vi "svfa_Check Data Valid [FFT] (N Ch).vi"(0 "scaled signals":waveform(dbl)[](array[waveform]), 2 "restart averaging (F)":bool, 7 "window":T2=1 items=["None"=0, "Hanning"=1, "Hamming"=2, "Blackman-Harris"=3, "Exact Blackman"=4, "Blackman"=5, "Flat Top"=6, "4 Term B-Harris "=7, "7 Term B-Harris"=8, "Low Sidelobe"=9, "Force"=64, "Exponential"=65, "Blackman Nuttall"=11, "Triangle"=30, "Bartlett-Hanning"=31, "Bohman"=32, "Parzen"=33, "Welch"=34, "Kaiser"=60, "Dolph-Chebyshev"=61, "Gaussian"=62], 9 "averaging parameters":T1={"averaging mode"=enum."No averaging", "weighting mode"=enum."Linear", "number of averages"=10, "linear mode"=enum."Auto restart"}, 11 "error in (no error)":errorcluster) -> (3 "restart averaging":bool, 4 "dup scaled signals":waveform(dbl)[](array[waveform]), 8 "dup window":T2=1 items=["None"=0, "Hanning"=1, "Hamming"=2, "Blackman-Harris"=3, "Exact Blackman"=4, "Blackman"=5, "Flat Top"=6, "4 Term B-Harris "=7, "7 Term B-Harris"=8, "Low Sidelobe"=9, "Force"=64, "Exponential"=65, "Blackman Nuttall"=11, "Triangle"=30, "Bartlett-Hanning"=31, "Bohman"=32, "Parzen"=33, "Welch"=34, "Kaiser"=60, "Dolph-Chebyshev"=61, "Gaussian"=62], 10 "dup averaging parameters":T1, 15 "error out":errorcluster)   [LabVIEW 2017]
doc: "returns errors on invalid parameters \nchecks for property changes (such as dt) and configuration changes (such as window), returns restart = TRUE on change"
uses:
  <vilib>/addons/_NISVFA/_Shared subVIs/Controls/svc_Window.ctl
  <vilib>/addons/_NISVFA/_Shared subVIs/Common/svc_Check for Waveform Parameter Continuity (no state).vi
  <vilib>/addons/_NISVFA/_Shared subVIs/Common/svc_Get SV Channel Info.vi
  <vilib>/addons/_NISVFA/_Shared subVIs/Common/svc_Engineering Units to Unit Label.vi
  <vilib>/addons/_NISVFA/_Shared subVIs/Common/svc_Unit Label to Engineering Units.vi
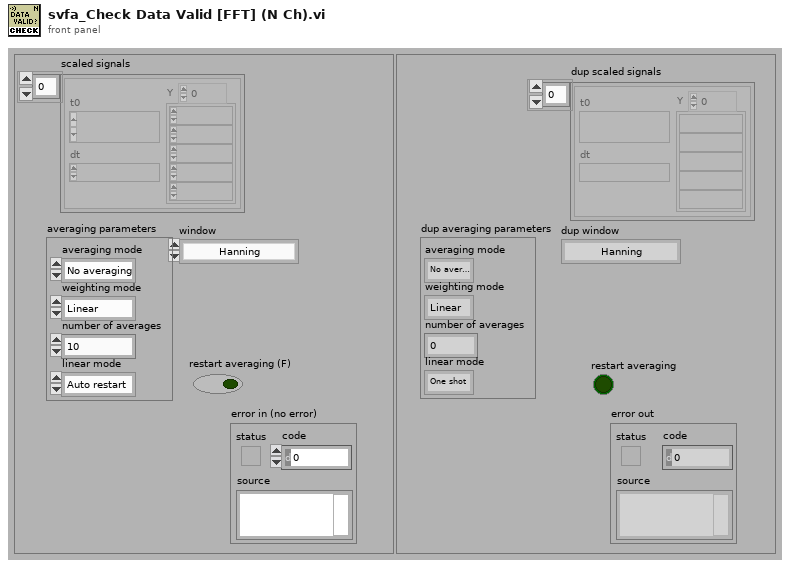
[diagram p1: front panel]
types:
  T1 = cluster{"averaging mode":enum16{"No averaging", "Vector averaging", "RMS averaging", "Peak hold"}, "weighting mode":enum16{"Linear", "Exponential"}, "number of averages":u32, "linear mode":enum16{"One shot", "Auto restart"}}
  T2 = typedef "svc_Window.ctl" = u32
  T3 = cluster{"dt equal":bool, "array length equal":bool, "number channels change":bool}
  T4 = cluster{"dt":bool, "t0 continuity":bool, "array length":bool, "channel info":bool, "name":bool}
  T5 = enum16{"No averaging", "Vector averaging", "RMS averaging", "Peak hold"}
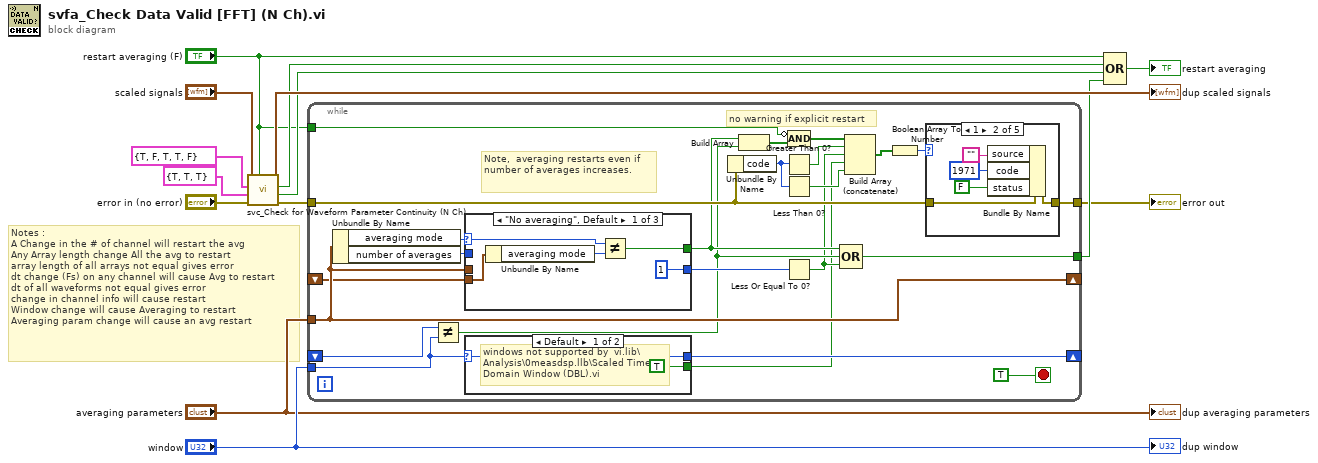
[diagram p0: block diagram]
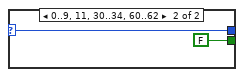
[diagram p2: hidden frame]
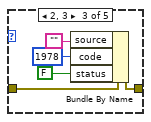
[diagram p4: hidden frame]
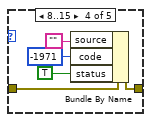
[diagram p5: hidden frame]
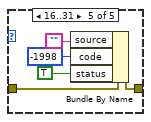
[diagram p6: hidden frame]
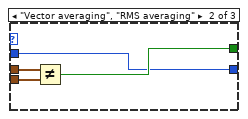
[diagram p7: hidden frame]
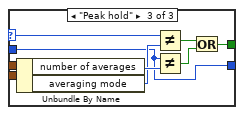
[diagram p8: hidden frame]
diagram:
  # "Notes : \nA Change in the # of channel will restart the avg\nAny Array length change All the avg to restart\narray length of all arrays not equal gives error\ndt change (Fs) on any channel will cause Avg to restart\ndt of all waveforms not equal gives error\nchange in channel info will cause restart\nWindow change will cause Averaging to restart\nAveraging param change will cause an avg restart"
  n1 = call <vilib>:"svc_Check for Waveform Parameter Continuity (N Ch).vi"("restart averaging (F)"="restart averaging (F)", "error in (no error)"="error in (no error)", "checks for multichannel parameters"=T3 {"dt equal"=TRUE, "array length equal"=TRUE, "number channels change"=TRUE}, "checks for channel parameter change"=T4 {"dt"=TRUE, "t0 continuity"=FALSE, "array length"=TRUE, "channel info"=TRUE, "name"=FALSE}, "scaled signal(s)"="scaled signals") -> ("error out"=w6:errorcluster, "multichannel parameter changed"=w9:bool, "waveform parameter changed"=w10:bool, "dup scaled signal(s)"=→"dup scaled signals":waveform(dbl)[])  [unwired: 3 out]
  n2 = while {
    tunnel: w6 -> [w23]
    tunnel: "restart averaging (F)" -> [w27]
    shift-right: [w16] -> _
    shift-left: _ -> [w37]
    tunnel: "window" -> [w17]
    shift-right: [w29] -> _
    shift-left: _ -> [w28]
    tunnel: "averaging parameters" -> [w29]
    tunnel: [w18] -> w4
    tunnel: [w22] -> w3
    stop <- TRUE stop-if-true
    # "Note,  averaging restarts even if number of averages increases."
    # "no warning if explicit restart"
    n3 = Unbundle By Name(w29) -> ("averaging mode"=w36:T5, "number of averages"=w35:u32)
    n4 = Not Equal?(x=w37, y=w17) -> (x != y?=w20:bool)
    n5 = case shown="\"No averaging\", Default" w36 {
      selector: w36 -> [w65 _ w76]
      tunnel: w29 -> [_ w71 _]
      tunnel: w28 -> [w68 w72 w75]
      tunnel: [w67 w70 w77] -> w21
      tunnel: w35 -> [_ w69 w73]
      tunnel: [u32 1 ("number of averages") w69 w73] -> w30
      frame "No averaging", Default {
        n6 = Unbundle By Name(w68) -> ("averaging mode"=w66:T5)
        n7 = Not Equal?(x=w65, y=w66) -> (x != y?=w67:bool)
      }
      frame "Vector averaging", "RMS averaging" {
        n8 = Not Equal?(x=w71, y=w72) -> (x != y?=w70:bool)
      }
      frame "Peak hold" {
        n9 = Unbundle By Name(w75) -> ("number of averages"=w80:u32, "averaging mode"=w74:T5)
        n10 = Not Equal?(x=w76, y=w74) -> (x != y?=w78:bool)
        n11 = Not Equal?(x=w73, y=w80) -> (x != y?=w79:bool)
        n12 = Or(x=w78, y=w79) -> (x .or. y?=w77:bool)
      }
    }
    n13 = case shown="Default" w17 {
      selector: w17 -> [w39 w41]
      tunnel: [TRUE FALSE] -> w15
      tunnel: [w39 w41] -> w16
      frame Default {
        # "windows not supported by  vi.lib\\Analysis\\0measdsp.llb\\Scaled Time Domain Window (DBL).vi"
      }
      frame 0..9, 11, 30..34, 60..62 {
      }
    }
    n14 = Unbundle By Name(w23) -> ("code"=w24:i32)
    n15 = Build Array(w21, w20) -> (w33:bool[])
    n16 = Greater Than 0?(x=w24) -> (x > 0?=w26:bool)
    n17 = Less Than 0?(x=w24) -> (x < 0?=w25:bool)
    n18 = Less Or Equal To 0?(x=w30) -> (x <= 0?=w19:bool)
    n19 = Compound Arithmetic op=AND(invert w27, w33) -> (w31:bool[])
    n20 = Compound Arithmetic op=OR(w21, w20, w19) -> (w18:bool)
    n21 = Build Array (concatenate)(w31, w26, w19, w15, w25) -> (w34:bool[])
    n22 = Boolean Array To Number(Boolean array=w34) -> (number=w32:u32)
    n23 = case shown="1" w32 {
      tunnel: w23 -> [w43 w45 w50 w55 w60]
      tunnel: [w43 w44 w49 w54 w59] -> w22
      frame 0, 4..7, 32..63, Default {
      }
      frame 1 {
        n24 = Bundle By Name(cluster=w45, "source"="", "code"=1971, "status"=FALSE) -> (w44:errorcluster)
      }
      frame 2, 3 {
        n25 = Bundle By Name(cluster=w50, "source"="", "code"=1978, "status"=FALSE) -> (w49:errorcluster)
      }
      frame 8..15 {
        n26 = Bundle By Name(cluster=w55, "source"="", "code"=-1971, "status"=TRUE) -> (w54:errorcluster)
      }
      frame 16..31 {
        n27 = Bundle By Name(cluster=w60, "source"="", "code"=-1998, "status"=TRUE) -> (w59:errorcluster)
      }
    }
  }
  "error out" <- w3
  n28 = Compound Arithmetic op=OR("restart averaging (F)", w10, w9, w4) -> (→"restart averaging":bool)
  "dup window" <- "window"
  "dup averaging parameters" <- "averaging parameters"
